vi "Obtain Request Events.vi"(8 "error in":errorcluster, 10 "Create New? (F)":bool) -> (0 "error out":errorcluster, 2 "Message Request Events":T1)   [LabVIEW 2024, in "Message.lvlib"]
doc: "This VI Obtains/Creates the Requests events that will be used for other modules to communicate with the module that owns this VI. These Requests events will be accessed only via Public API methods for this module.\n\n<b>NOTE</b>: The contents of this VI are automatically generated and modified by the <b>Tools > DQMH Consortium > DQMH</b> utilities. Consider using those utilities instead of making your own modifications to this VI.\n_____\nBased on DQMH Dev Tools: Project Template 7.1.0.1503."
uses:
  Message.lvlib
  Request Events--cluster.ctl
  Stop Argument--cluster.ctl
  Show Panel Argument--cluster.ctl
  Hide Panel Argument--cluster.ctl
  Show Diagram Argument--cluster.ctl
  Get Module Execution Status Argument--cluster.ctl
  Draw FP in Subpanel Argument--cluster.ctl
  Remove From Subpanel Argument--cluster.ctl
  Set Message Argument--cluster.ctl
  Append String Argument--cluster.ctl
  Set Text Font Settings Argument--cluster.ctl
  <vilib>/Utility/miscctls.llb/LVFontTypeDef.ctl
panel:
  # "NOTE: The contents of this VI are automatically generated and modified by the Tools > DQMH Consortium > DQMH utilities. Consider using those utilities instead of making your own modifications to this VI."
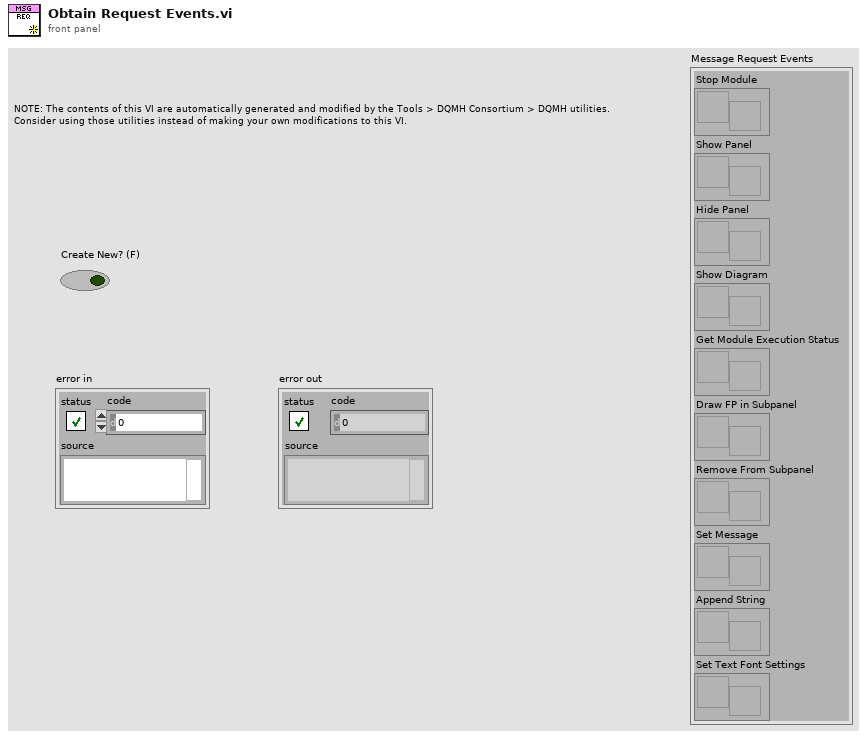
[diagram p1: front panel]
types:
  T1 = typedef "Message.lvlib/Request Events--cluster.ctl" = cluster{"Stop Module":refnum<user-event>, "Show Panel":refnum<user-event>, "Hide Panel":refnum<user-event>, "Show Diagram":refnum<user-event>, "Get Module Execution Status":refnum<user-event>, "Draw FP in Subpanel":refnum<user-event>, "Remove From Subpanel":refnum<user-event>, "Set Message":refnum<user-event>, "Append String":refnum<user-event>, "Set Text Font Settings":refnum<user-event>}
  T2 = typedef "Message.lvlib/Set Text Font Settings Argument--cluster.ctl" = cluster{"Module ID":i32, "Text.Font":T3}
  T3 = typedef "LVFontTypeDef.ctl" = cluster{"Font Name":string, "Size":u16, "Bold":bool, "Italic":bool, "Underline":bool, "Strikeout":bool, "Color":u32}
  T4 = typedef "Message.lvlib/Append String Argument--cluster.ctl" = cluster{"Module ID":i32, "String":string}
  T5 = typedef "Message.lvlib/Set Message Argument--cluster.ctl" = cluster{"Module ID":i32, "Message":string}
  T6 = typedef "Message.lvlib/Remove From Subpanel Argument--cluster.ctl" = cluster{"Module ID":i32, "Boolean":bool}
  T7 = typedef "Message.lvlib/Draw FP in Subpanel Argument--cluster.ctl" = cluster{"Module ID":i32, "Sub Panel":refnum<vi>}
  T8 = typedef "Message.lvlib/Get Module Execution Status Argument--cluster.ctl" = cluster{"Module ID":i32, "Running?":bool}
  T9 = typedef "Message.lvlib/Show Diagram Argument--cluster.ctl" = cluster{"Module ID":i32, "Debug?":bool}
  T10 = typedef "Message.lvlib/Show Panel Argument--cluster.ctl" = cluster{"Module ID":i32, "Show Panel?":bool}
  T11 = typedef "Message.lvlib/Hide Panel Argument--cluster.ctl" = cluster{"Module ID":i32, "Hide Panel?":bool}
  T12 = typedef "Message.lvlib/Stop Argument--cluster.ctl" = cluster{"Module ID":i32, "Origin":string, "Exit via Stop Module Req?":bool, "Wait for Module to stop?":bool}
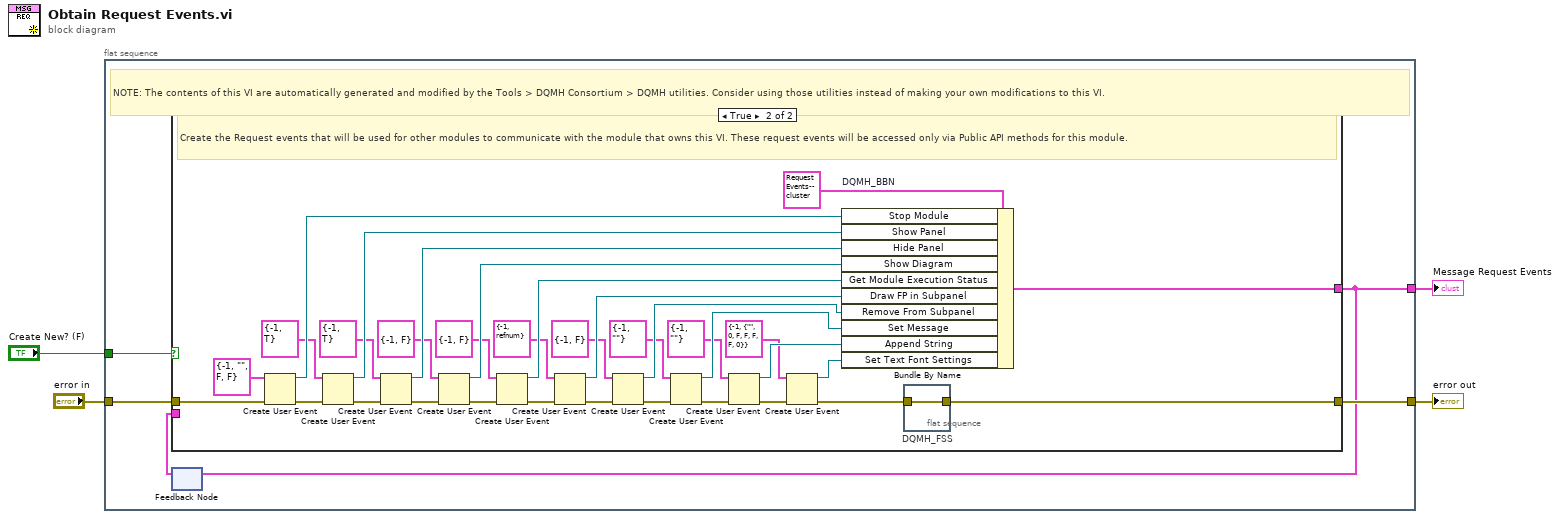
[diagram p0: block diagram]
diagram:
  n1 = flat-sequence {
    tunnel: [w9] -> w4
    tunnel: "error in" -> [w8]
    tunnel: [w6] -> w2
    tunnel: "Create New? (F)" -> [w5]
    frame #0 {
      # "NOTE: The contents of this VI are automatically generated and modified by the Tools > DQMH Consortium > DQMH utilities. Consider using those utilities instead of making your own modifications to this VI."
      n2 = feedback #1() -> (w7:T1)  [unwired: 1 in]
      n3 = case shown="True" w5 {
        tunnel: [w10 w33] -> w9
        tunnel: w8 -> [w10 w45]
        tunnel: [w11 w42] -> w6
        tunnel: w7 -> [w11 _]
        frame False {
        }
        frame True {
          # "Create the Request events that will be used for other modules to communicate with the module that owns this VI. These request events will be accessed only via Public API methods for this module."
          n4 = Create User Event(user event datatype=T12 {"Module ID"=-1, "Origin"="", "Exit via Stop Module Req?"=FALSE, "Wait for Module to stop?"=FALSE} ("Stop Argument"), error in=w45) -> (user event=w43:refnum<user-event>, error out=w40:errorcluster)
          n5 = Create User Event(user event datatype=T10 {"Module ID"=-1, "Show Panel?"=TRUE} ("Show Panel Argument"), error in=w40) -> (user event=w39:refnum<user-event>, error out=w37:errorcluster)
          n6 = Create User Event(user event datatype=T11 {"Module ID"=-1, "Hide Panel?"=TRUE} ("Hide Panel"), error in=w37) -> (user event=w36:refnum<user-event>, error out=w35:errorcluster)
          n7 = Create User Event(user event datatype=T9 {"Module ID"=-1, "Debug?"=FALSE} ("Show Diagram Argument"), error in=w35) -> (user event=w31:refnum<user-event>, error out=w32:errorcluster)
          n8 = Create User Event(user event datatype=T8 {"Module ID"=-1, "Running?"=FALSE} ("Get Module Execution Status Argument"), error in=w32) -> (user event=w28:refnum<user-event>, error out=w29:errorcluster)
          n9 = Create User Event(user event datatype=T7 {"Module ID"=-1, "Sub Panel"=refnum} ("Draw FP in Subpanel Argument"), error in=w29) -> (user event=w25:refnum<user-event>, error out=w26:errorcluster)
          n10 = Create User Event(user event datatype=T6 {"Module ID"=-1, "Boolean"=FALSE} ("Remove From Subpanel Argument"), error in=w26) -> (user event=w22:refnum<user-event>, error out=w23:errorcluster)
          n11 = Create User Event(user event datatype=T5 {"Module ID"=-1, "Message"=""} ("Set Message Argument"), error in=w23) -> (user event=w19:refnum<user-event>, error out=w20:errorcluster)
          n12 = Create User Event(user event datatype=T4 {"Module ID"=-1, "String"=""} ("Append String Argument"), error in=w20) -> (user event=w16:refnum<user-event>, error out=w17:errorcluster)
          n13 = Create User Event(user event datatype=T2 {"Module ID"=-1, "Text.Font"={"Font Name"="", "Size"=0, "Bold"=FALSE, "Italic"=FALSE, "Underline"=FALSE, "Strikeout"=FALSE, "Color"=0}} ("Set Text Font Settings Argument"), error in=w17) -> (user event=w13:refnum<user-event>, error out=w14:errorcluster)
          n14 = Bundle By Name "DQMH_BBN"(cluster=T1 {"Stop Module"=refnum, "Show Panel"=refnum, "Hide Panel"=refnum, "Show Diagram"=refnum, "Get Module Execution Status"=refnum, "Draw FP in Subpanel"=refnum, "Remove From Subpanel"=refnum, "Set Message"=refnum, "Append String"=refnum, "Set Text Font Settings"=refnum} ("output cluster"), "Stop Module"=w43, "Show Panel"=w39, "Hide Panel"=w36, "Show Diagram"=w31, "Get Module Execution Status"=w28, "Draw FP in Subpanel"=w25, "Remove From Subpanel"=w22, "Set Message"=w19, "Append String"=w16, "Set Text Font Settings"=w13) -> (w42:T1)
          n15 = flat-sequence "DQMH_FSS" {
            tunnel: w14 -> [w46]
            tunnel: [w46] -> w33
            frame #0 {
            }
          }
        }
      }
      n16 = feedback-in #1(w6) -> ()
    }
  }
  "Message Request Events" <- w2
  "error out" <- w4
